vi "Write Translator.vi"(8 "error in (no error)":errorcluster, 10 "Messenging.lvlib:Translator.lvclass":refnum<class "Translator.lvclass">, 11 "Observer.lvclass in":refnum<class "Observer.lvclass">) -> (0 "error out":errorcluster, 3 "Observer.lvclass out":refnum<class "Observer.lvclass">)   [LabVIEW 2011, in "Messenging.lvlib" / "Observer.lvclass"]
uses:
  Observer.lvclass
  Message Translation/Translator/Translator.lvclass
  Observer.lvclass/Observer.ctl
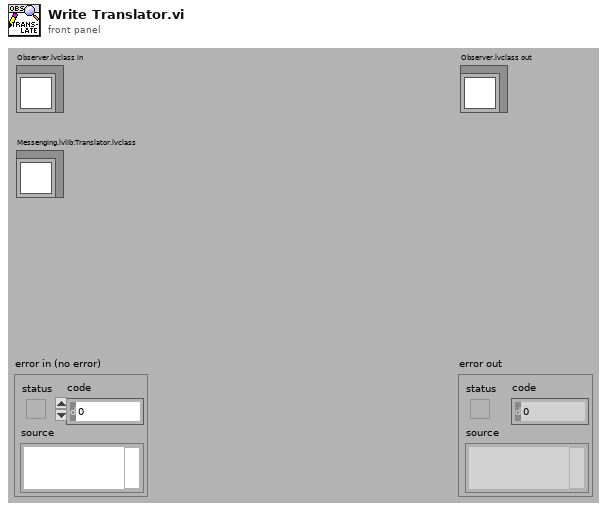
[diagram p1: front panel]
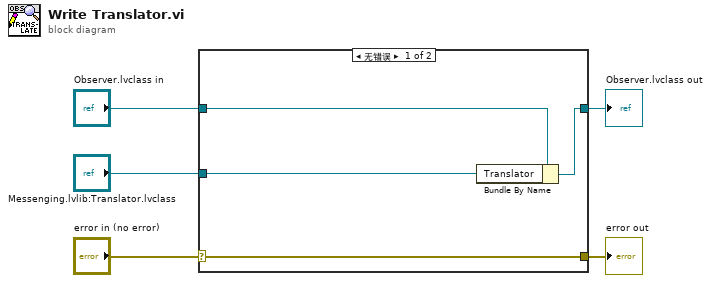
[diagram p0: block diagram]
diagram:
  n1 = case shown="无错误" "error in (no error)" {
    selector: "error in (no error)" -> [w9 w10]
    tunnel: [w9 w10] -> w4
    tunnel: [w7 w11] -> w2
    tunnel: "Observer.lvclass in" -> [w8 w11]
    tunnel: "Messenging.lvlib:Translator.lvclass" -> [w6 _]
    frame No Error {
      n2 = Bundle By Name(cluster=w8, "Translator"=w6) -> (w7:refnum<class "Observer.lvclass">)
    }
    frame Error {
    }
  }
  "error out" <- w4
  "Observer.lvclass out" <- w2
